vi "Target Encoder Angle from Voltages.vi"(10 "Encoder Voltage B (V)":dbl, 11 "Encoder Voltage A (V)":dbl) -> (3 "Encoder Angle (deg)":dbl)   [LabVIEW 2018, in "COBRA Measurement and Filtering Library.lvlib"]
uses:
  COBRA Measurement and Filtering Library.lvlib
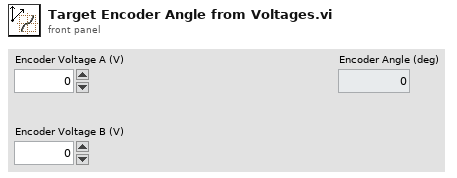
[diagram p1: front panel]
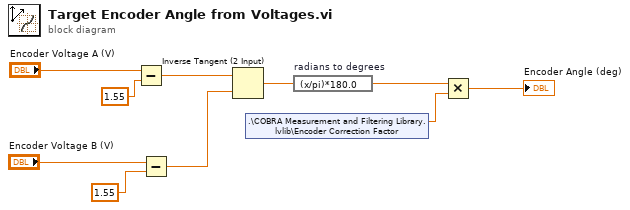
[diagram p0: block diagram]
diagram:
  n1 = Subtract(x="Encoder Voltage A (V)", y=1.55) -> (x-y=w7:dbl)
  n2 = Subtract(x="Encoder Voltage B (V)", y=1.55) -> (x-y=w6:dbl)
  n3 = Inverse Tangent (2 Input)(1:w6, 2:w7) -> (0:w10:dbl)
  n4 = shared-variable ".\\COBRA Measurement and Filtering Library.lvlib\\Encoder Correction Factor"() -> (w2:dbl)  [unwired: 1 in, 1 out]
  n5 = expression code="(x/pi)*180.0" "radians to degrees"(w10) -> (w5:dbl)
  n6 = Multiply(x=w5, y=w2) -> (x*y=→"Encoder Angle (deg)":dbl)
